vi "CloseSwitch.vi"(2 "error in (no error)":errorcluster, 3 "Switch ID":i32=1020 format="%_4g") -> (0 "error out":errorcluster)   [LabVIEW 2009]
doc: "Closes switch with speciafied ID"
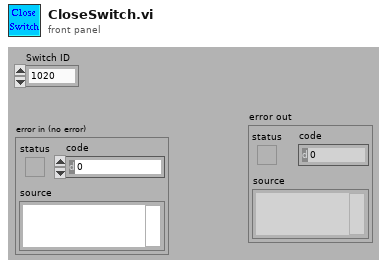
[diagram p1: front panel]
types:
  T1 = enum16{"N1911A", "Siggen", "34980a", "E4418B", "Rvp8"}
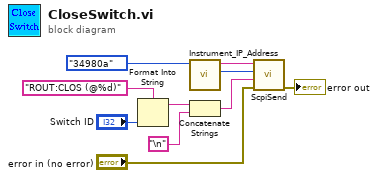
[diagram p0: block diagram]
diagram:
  n1 = Format Into String(format string="ROUT:CLOS (@%d)", "Switch ID") -> (resulting string=w7:string)  [unwired: 2 in, 1 out]
  n2 = call "Instrument_IP_Address.vi"("Instrument"=T1."34980a") -> ("Port"=w2:u16, "IP Address"=w3:string)  [unwired: 9 in]
  n3 = Concatenate Strings(w7, "\n") -> (w6:string)
  n4 = call "ScpiSend.vi"("error in (no error)"="error in (no error)", "Command"=w6, "TCP port"=w2, "IP Address"=w3) -> ("error out"=→"error out":errorcluster)  [unwired: 7 in]
